vi "Interpolate_dataview.vi"(8 "Y-column names":string[](array[string])=["mr"], 10 "column extension":string[](array[string])=["022", "016"], 11 "Graph array":cluster{"output":dbl[], "output":dbl[]}[](array[cluster])=[{"output"=array[5704 elements], "output"=array[5704 elements]}, {"output"=array[27359 elements], "output"=array[27359 elements]}]) -> ()   [LabVIEW 2025]
uses:
  <vilib>/gmath/NI_Gmath.lvlib
panel:
  in  "number format":string="%5.5f"
  in  "column delimitter":enum16{"tab", "comma (,)", "space", "write in"}(ring)
  in  "x-wave delimiter":u16(ring)=1 items=["tab", "carriage return", "space"]
  in  "interpolation x-wave":string
  in  "make x-wave":bool caption="x-wave in the worksheet"
  in  "y-axis":bool
  in  "x-axis":bool
  in  "pts #":i32=100
  in  "reduce pts (before interpolate)":bool
  out "min value":dbl
  out "max value":dbl
  in  "min":dbl=2.0 min=0.0 format="%.2f"
  in  "interpolation method":i32(ring)=1 items=["nearest", "linear", "spline", "cubic Hermite", "Lagrange"]
  out "y-column name":string
  in  "smooth":bool
  in  "smooth factor":i32=121
  in  "iteration Number":i32=2
  in  "interpolation size":u16=2 min=2 step=1
  in  "max":dbl=2.0 min=0.0 format="%.2f"
  in  "export":T1(ring)=enum."write to clipboard"
  out "raw data":cluster{"output":dbl[], "smoothed":dbl[]}[](graph)
  in  "stop":bool=TRUE
  in  "export data":bool
  # "Fitting is done for the range given by 'Bbkg init' and 'Bbkg final'.\nBackground curve is extended to the range give by 'B init' and 'B final'.\nFFT is done in the range given by 'B init' and 'B final'."
  # "Log scale?"
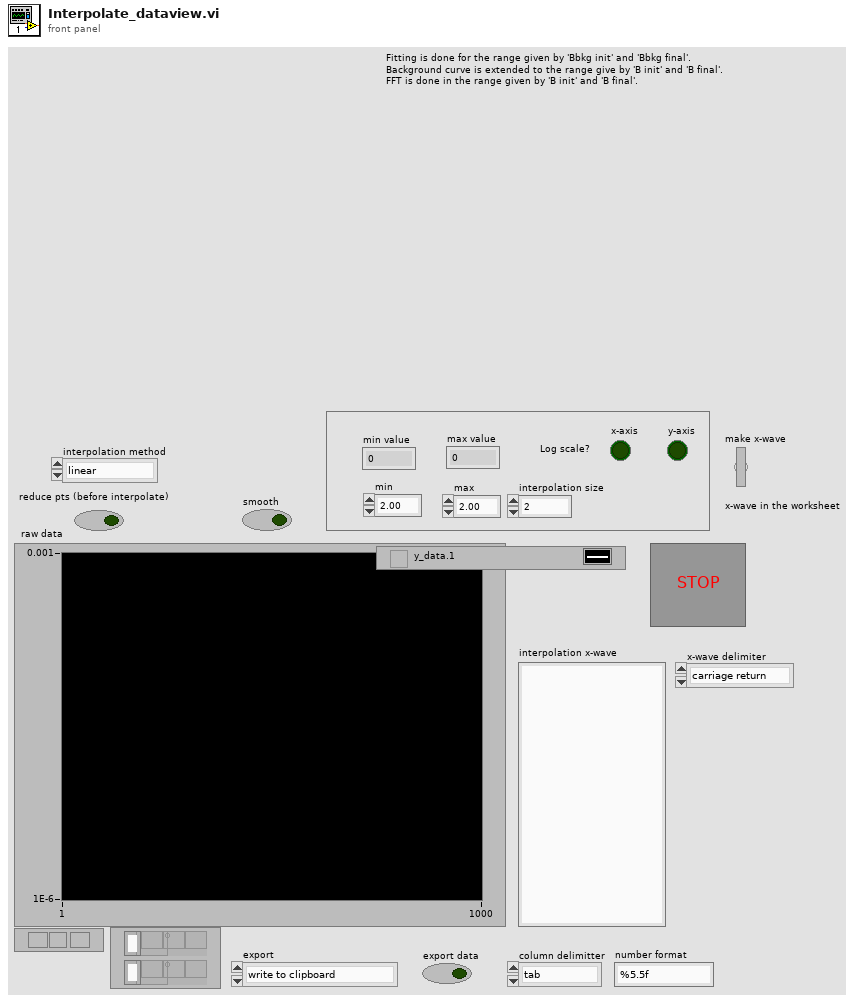
[diagram p1: front panel]
types:
  T1 = enum16{"Save as Ascill file", "write to clipboard", "write to Igor ITX file"}
  T2 = enum16{"Save as Ascill file", "write to clipboard", "do not export"}
  T3 = cluster{"cleaned array":dbl[], "cleaned array":dbl[]}
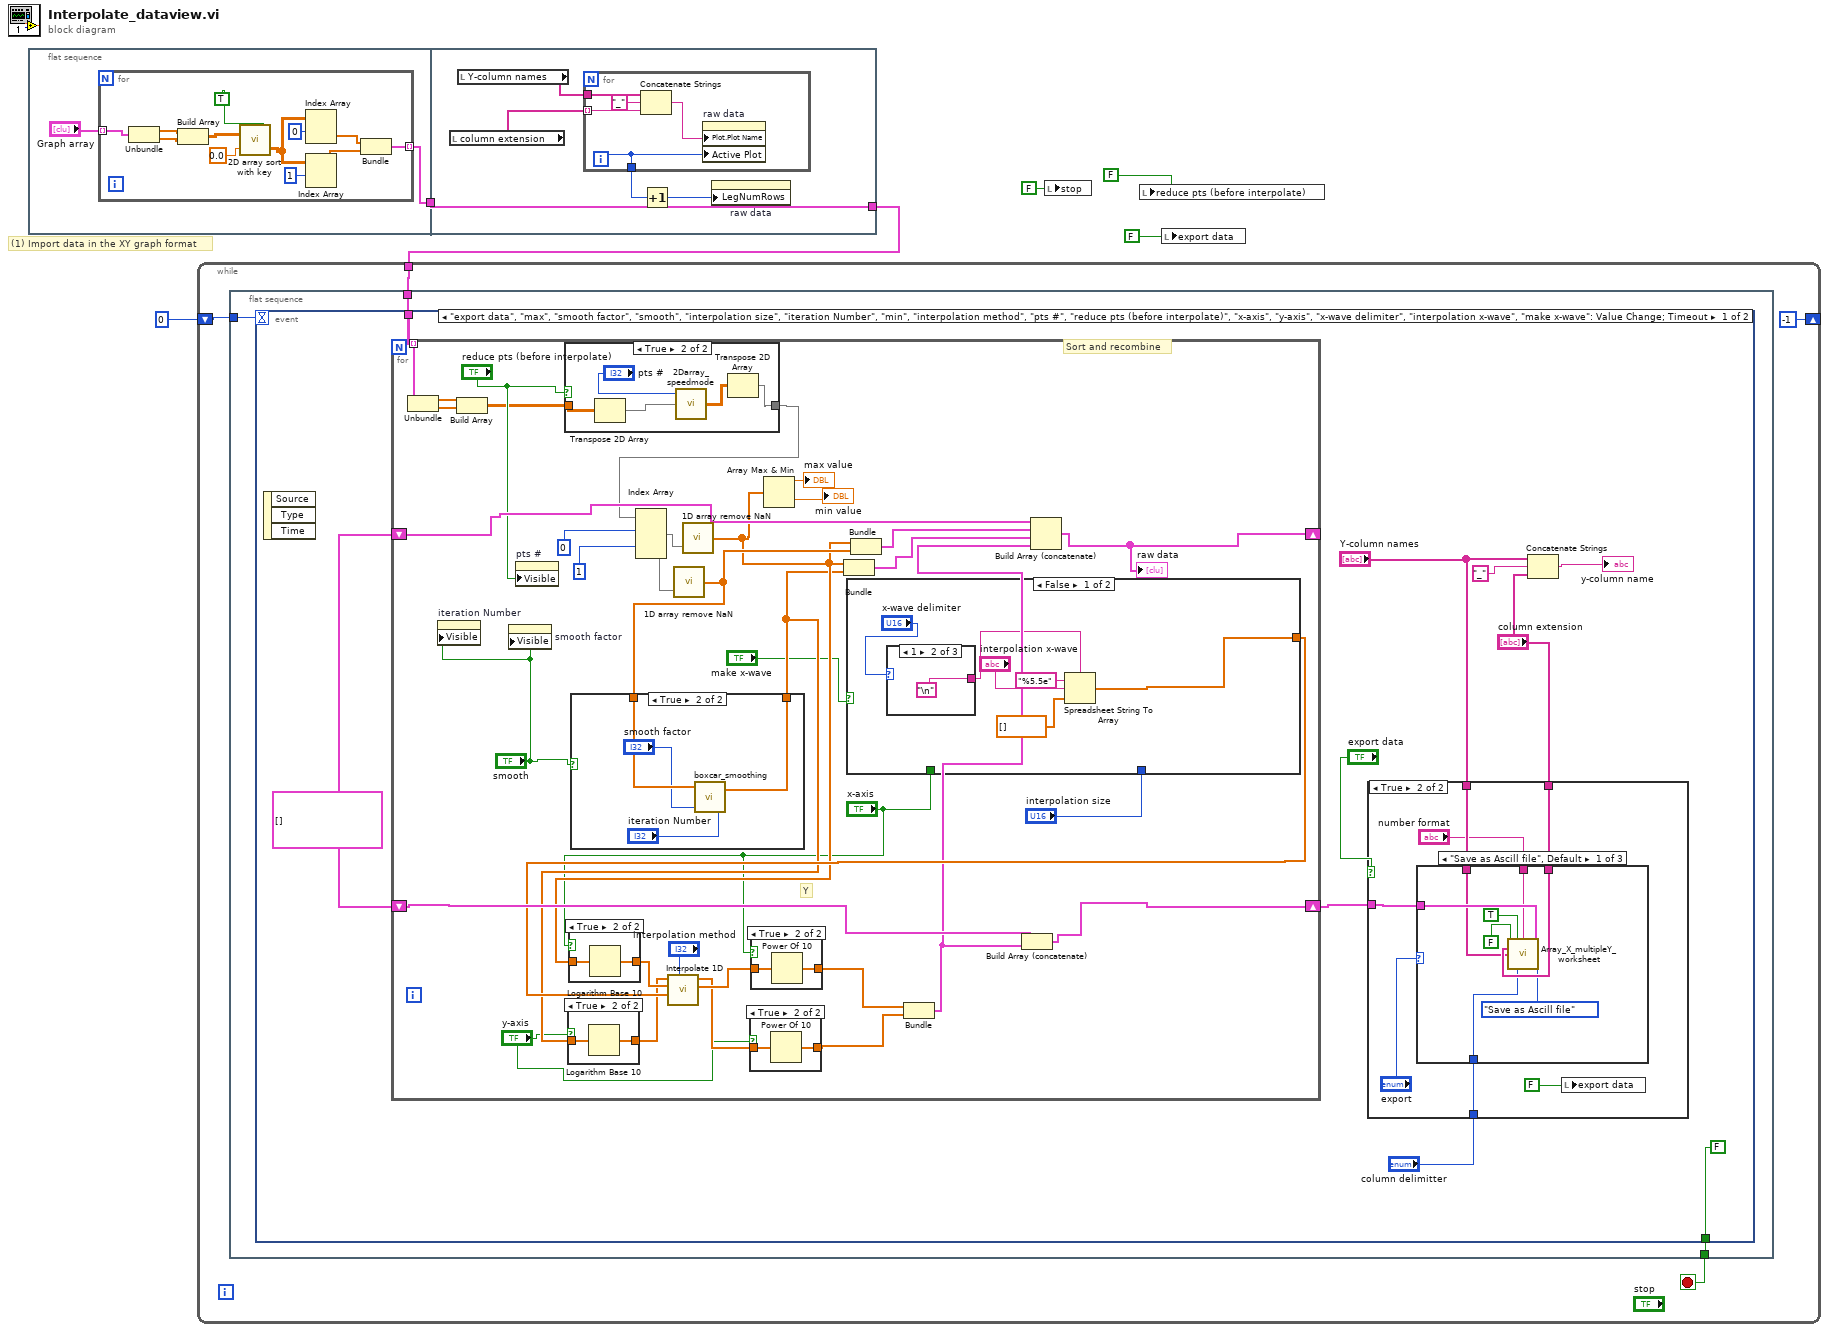
[diagram p0: block diagram]
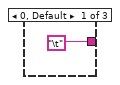
[diagram p2: hidden frame]
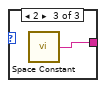
[diagram p3: hidden frame]
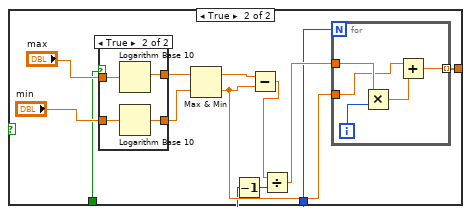
[diagram p4: hidden frame]
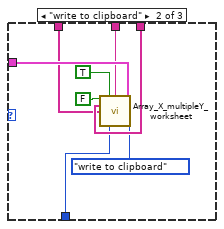
[diagram p13: hidden frame]
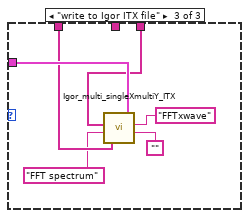
[diagram p14: hidden frame]
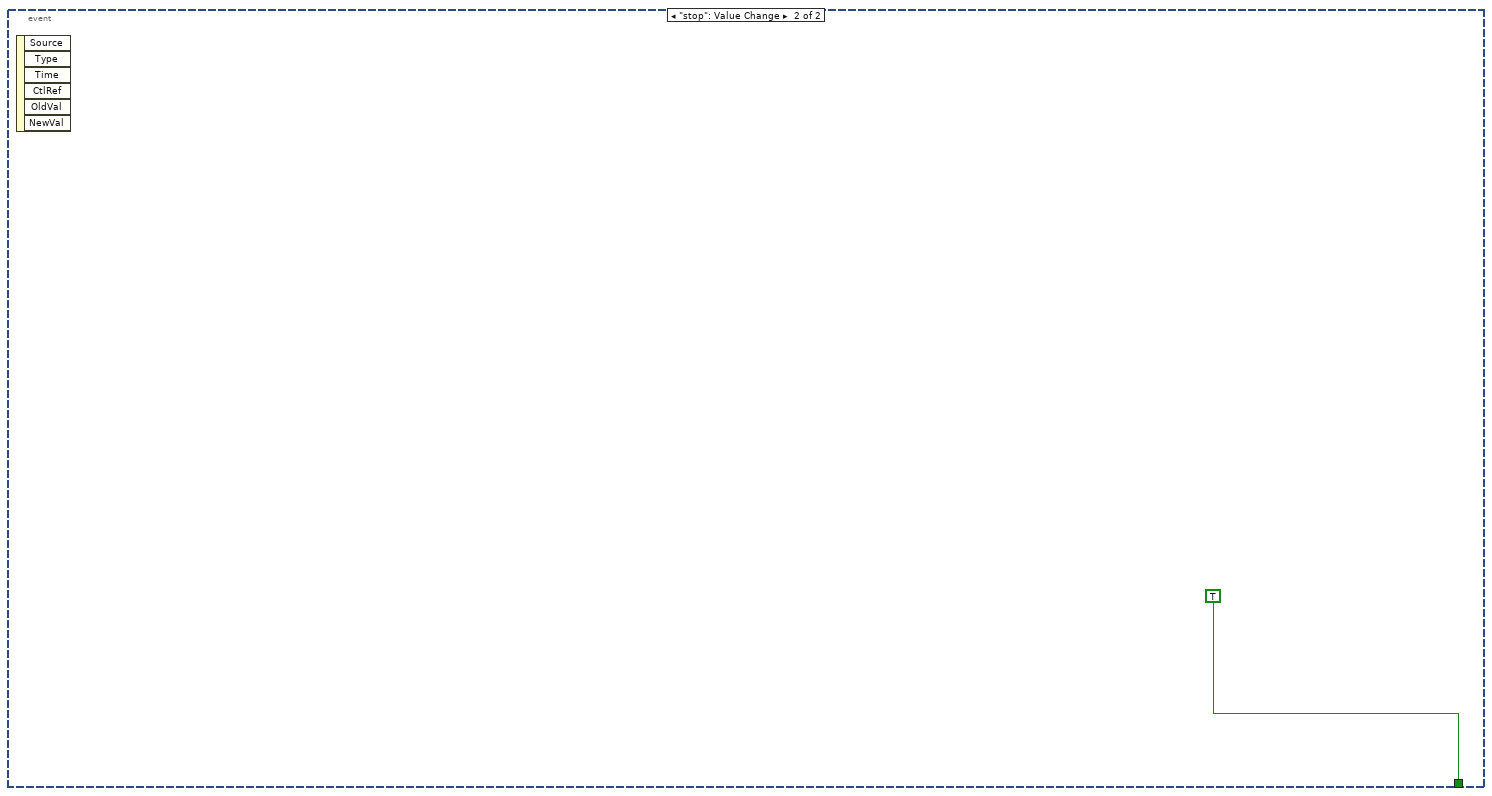
[diagram p15: hidden frame]
diagram:
  # "(1) Import data in the XY graph format"
  n1 = flat-sequence {
    tunnel: [w8] -> w2
    tunnel: [w25] -> w1
    tunnel: w2 -> [w25]
    frame #0 {
      n2 = for {
        tunnel: "Graph array" -> [w20] mode=indexing
        tunnel: [w9] -> w8 mode=indexing
        n3 = Unbundle(w20) -> ("output"=w18:dbl[], "output"=w17:dbl[])
        n4 = Build Array(w18, w17) -> (w16:dbl[][])
        n5 = call "2D array sort with key.vi"("ascending"=TRUE, "key row"=0.0, "input"=w16) -> ("output"=w14:dbl[][])
        n6 = Index Array(array=w14, index (row)=0) -> (element=w11:dbl[])  [unwired: 1 in]
        n7 = Index Array(array=w14, index (row)=1) -> (element=w10:dbl[])  [unwired: 1 in]
        n8 = Bundle("output"=w11, "output"=w10) -> (w9:cluster{"output":dbl[], "output":dbl[]})  [unwired: 1 in]
      }
    }
    frame #1 {
      n9 = local read "column extension"() -> (w23:string[])
      n10 = local read "Y-column names"() -> (w24:string[])
      n11 = for {
        tunnel: w24 -> [w29]
        tunnel: w23 -> [w28] mode=indexing
        tunnel: [w26] -> w22
        i -> [w26]
        n12 = Concatenate Strings(w29, "_" ("column_extension"), w28) -> (w27:string)
        n13 = property on="raw data" class="XYGraph (strict)"("Plot.Plot Name"=w27, "Active Plot"=w26) -> ()  [unwired: 2 in, 2 out]
      }
      n14 = Increment(x=w22) -> (x+1=w21:i32)
      n15 = property on="raw data" class="XYGraph (strict)"("LegNumRows"=w21) -> ()  [unwired: 2 in, 2 out]
    }
  }
  n16 = while {
    tunnel: w1 -> [w34]
    shift-right: [-1] -> _
    shift-left: 0 -> [w31]
    stop <- w33 stop-if-true
    n17 = flat-sequence {
      tunnel: w34 -> [w37]
      tunnel: [w36] -> w33
      tunnel: w31 -> [w35]
      frame #0 {
        n18 = event shown="[0] \"export data\", \"max\", \"smooth factor\", \"smooth\", \"interpolation size\", \"iteration Number\", \"min\", \"interpolation method\", \"pts #\", \"reduce pts (before interpolate)\", \"x-axis\", \"y-axis\", \"x-wave delimiter\", \"interpolation x-wave\", \"make x-wave\": Value Change;  Timeout" {
          selector: _ -> [_ _]
          dyn-events: _ -> [_ _]
          timeout: w35 -> [_ _]
          tunnel: w37 -> [w46 _]
          tunnel: [FALSE ("stop (press twice)") TRUE ("stop (press twice)")] -> w36
          event "export data", "max", "smooth factor", "smooth", "interpolation size", "iteration Number", "min", "interpolation method", "pts #", "reduce pts (before interpolate)", "x-axis", "y-axis", "x-wave delimiter", "interpolation x-wave", "make x-wave": Value Change; Timeout {
            w44 = cluster{"all rows":sgl[], "all rows":sgl[]}[] []
            n19 = event-data() -> ()  [unwired: 1 in, 3 out]
            n20 = for {
              shift-right: [w77] -> w43
              shift-left: w44 -> [w78]
              tunnel: w46 -> [w82] mode=indexing
              shift-right: [w76] -> _
              shift-left: w44 -> [w79]
              # "Y"
              # "Sort and recombine"
              n21 = Unbundle(w82) -> ("output"=w81:dbl[], "output"=w80:dbl[])
              n22 = property on="iteration Number" class="DigNum (strict)"("Visible"="smooth") -> ()  [unwired: 2 in, 2 out]
              n23 = Build Array(w81, w80) -> (w59:dbl[][])
              n24 = property on="smooth factor" class="DigNum (strict)"("Visible"="smooth") -> ()  [unwired: 2 in, 2 out]
              n25 = property on="pts #" class="DigNum (strict)"("Visible"="reduce pts (before interpolate)") -> ()  [unwired: 2 in, 2 out]
              n26 = case shown="True" "reduce pts (before interpolate)" {
                tunnel: w59 -> [w127 w131]
                tunnel: [w127 w128] -> w63
                frame False {
                }
                frame True {
                  n27 = Transpose 2D Array(2D array=w131) -> (transposed array=w130:dbl[][])
                  n28 = call "2Darray_speedmode.vi"("original 2D array"=w130, "# of rows"="pts #") -> ("reduced 2D array"=w129:dbl[][])  [unwired: 1 in]
                  n29 = Transpose 2D Array(2D array=w129) -> (transposed array=w128:dbl[][])
                }
              }
              n30 = Index Array(array=w63, index (row) #1=0 ("disabled index (col)"), index (row) #2=1 ("index (col)")) -> (element #1=w65:dbl[], element #2=w61:dbl[])  [unwired: 2 in]
              n31 = call "1D array remove NaN.vi"("Array input"=w61) -> ("cleaned array"=w60:dbl[])  [unwired: 1 in]
              n32 = case shown="True" "smooth" {
                tunnel: w60 -> [w133 w137]
                tunnel: [w133 w136] -> w56
                frame False {
                }
                frame True {
                  n33 = call "boxcar_smoothing.vi"("iteration Number"="iteration Number", "smooth factor"="smooth factor", "raw data"=w137) -> ("smoothed"=w136:dbl[])  [unwired: 1 in]
                }
              }
              n34 = case shown="True" "y-axis" {
                tunnel: w56 -> [w121 w123]
                tunnel: [w121 w122] -> w55
                frame False {
                }
                frame True {
                  n35 = Logarithm Base 10(1:w123) -> (0:w122:dbl[])
                }
              }
              n36 = call "1D array remove NaN.vi"("Array input"=w65) -> ("cleaned array"=w58:dbl[])  [unwired: 1 in]
              n37 = case shown="True" "x-axis" {
                tunnel: w58 -> [w124 w126]
                tunnel: [w124 w125] -> w57
                frame False {
                }
                frame True {
                  n38 = Logarithm Base 10(1:w126) -> (0:w125:dbl[])
                }
              }
              n39 = Array Max & Min(array=w58) -> (max value=→"max value":dbl, min value=→"min value":dbl)  [unwired: 2 out]
              n40 = Bundle("cleaned array"=w58, "smoothed"=w56) -> (w67:cluster{"cleaned array":dbl[], "smoothed":dbl[]})  [unwired: 1 out]
              n41 = case shown="False" "make x-wave" {
                tunnel: "interpolation size" -> [_ w99]
                tunnel: [w83 w97] -> w66
                tunnel: "x-axis" -> [_ w92]
                frame False {
                  n42 = case shown="1" "x-wave delimiter" {
                    tunnel: ["\t" "\n" w91] -> w84
                    frame 0, Default {
                    }
                    frame 1 {
                    }
                    frame 2 {
                      n43 = call <vilib>:"Space Constant.vi"() -> ("String"=w91:string)
                    }
                  }
                  n44 = Spreadsheet String To Array(delimiter (Tab)=w84, format string="%5.5e", spreadsheet string="interpolation x-wave", array type (2D Dbl)=dbl[] []) -> (array=w83:dbl[])
                }
                frame True {
                  n45 = case shown="True" w92 {
                    tunnel: "max" -> [w105 w109]
                    tunnel: "min" -> [w104 w108]
                    tunnel: [w105 w107] -> w94
                    tunnel: [w104 w106] -> w93
                    frame False {
                    }
                    frame True {
                      n46 = Logarithm Base 10(1:w109) -> (0:w107:dbl)
                      n47 = Logarithm Base 10(1:w108) -> (0:w106:dbl)
                    }
                  }
                  n48 = Max & Min(x=w94, y=w93) -> (max(x,y)=w103:dbl, min(x,y)=w101:dbl)
                  n49 = Decrement(x=w99) -> (x-1=w98:u16)
                  n50 = Subtract(x=w103, y=w101) -> (x-y=w102:dbl)
                  n51 = Divide(x=w102, y=w98) -> (x/y=w100:dbl)
                  n52 = for {
                    N: w99 -> [_]
                    tunnel: [w114] -> w97 mode=indexing
                    tunnel: w101 -> [w110]
                    tunnel: w100 -> [w111]
                    i -> [w113]
                    n53 = Multiply(x=w111, y=w113) -> (x*y=w112:dbl)
                    n54 = Add(x=w110, y=w112) -> (x+y=w114:dbl)
                  }
                }
              }
              n55 = call <vilib>:"Interpolate 1D.vi"("method"="interpolation method", "xi"=w66, "X"=w57, "Y"=w55) -> ("xi used"=w54:dbl[], "yi"=w51:dbl[])  [unwired: 5 in, 1 out]
              n56 = case shown="True" "y-axis" {
                tunnel: w51 -> [w115 w117]
                tunnel: [w115 w116] -> w52
                frame False {
                }
                frame True {
                  n57 = Power Of 10(x=w117) -> (10^x=w116:dbl[])
                }
              }
              n58 = case shown="True" "x-axis" {
                tunnel: w54 -> [w118 w120]
                tunnel: [w118 w119] -> w53
                frame False {
                }
                frame True {
                  n59 = Power Of 10(x=w120) -> (10^x=w119:dbl[])
                }
              }
              n60 = Bundle("cleaned array"=w58, "cleaned array"=w60) -> (w72:T3)  [unwired: 1 out]
              n61 = Bundle("xi used"=w53, "yi"=w52) -> (w62:cluster{"xi used":dbl[], "yi":dbl[]})  [unwired: 1 out]
              n62 = Build Array (concatenate)(w78, w62) -> (w77:cluster{"xi used":dbl[], "yi":dbl[]}[])
              n63 = Build Array (concatenate)(w79, w72, w67, w62) -> (w76:cluster{"xi used":dbl[], "yi":dbl[]}[])
              "raw data" <- w76
            }
            n64 = case shown="True" "export data" {
              tunnel: w43 -> [_ w143]
              tunnel: "Y-column names" -> [_ w141]
              tunnel: "column extension" -> [_ w140]
              tunnel: "column delimitter" -> [_ w139]
              frame False {
              }
              frame True {
                n65 = case shown="\"Save as Ascill file\", Default" "export" {
                  tunnel: w143 -> [w152 w160 w166]
                  tunnel: w140 -> [w150 w158 w165]
                  tunnel: w141 -> [w149 w157 w164]
                  tunnel: w139 -> [w146 w154 _]
                  tunnel: "number format" -> [w145 w153 _]
                  frame "Save as Ascill file", Default {
                    n66 = call "Array_X_multipleY_worksheet.vi"("Sort?"=FALSE, "same x-data"=TRUE, "number format"=w145, "graph file"=w152, "column extension"=w150, "Y-column names"=w149, "export"=T2."Save as Ascill file", "column delimitter"=w146) -> ()  [unwired: 6 in, 2 out]
                  }
                  frame "write to clipboard" {
                    n67 = call "Array_X_multipleY_worksheet.vi"("Sort?"=FALSE, "same x-data"=TRUE, "number format"=w153, "graph file"=w160, "column extension"=w158, "Y-column names"=w157, "export"=T2."write to clipboard", "column delimitter"=w154) -> ()  [unwired: 6 in, 2 out]
                  }
                  frame "write to Igor ITX file" {
                    n68 = call "Igor_multi_singleXmultiY_ITX.vi"("message"="", "x-column name"="FFTxwave", "graph file"=w166, "Y-column names"=w164, "window name"="FFT spectrum", "column extension"=w165) -> ()  [unwired: 1 in, 1 out]
                  }
                }
                n69 = local write "export data"(FALSE ("export spectrum")) -> ()
              }
            }
            n70 = Concatenate Strings("Y-column names", "_" ("column_extension"), "column extension") -> (→"y-column name":string)
          }
          event "stop": Value Change {
            n71 = event-data() -> ()  [unwired: 1 in, 6 out]
          }
        }
      }
    }
  }
  n72 = local write "stop"(FALSE ("stop")) -> ()
  n73 = local write "reduce pts (before interpolate)"(FALSE ("reduce pts")) -> ()
  n74 = local write "export data"(FALSE ("export spectrum")) -> ()
